vi "Get-selected-motors.vi"(8 "error in (no error)":errorcluster, 11 "Object ref in":T1) -> (0 "error out":errorcluster, 2 "Active?":bool[](array[boolean]), 3 "Object ref out":T1)   [LabVIEW 2013, in "PowderDeposition.lvlib" / "PD-Main.lvclass"]
uses:
  PD-Main.lvclass
  Object-reference.ctl
  PD-Main.lvclass/PD-Main.ctl
  Read Motors-selection.vi
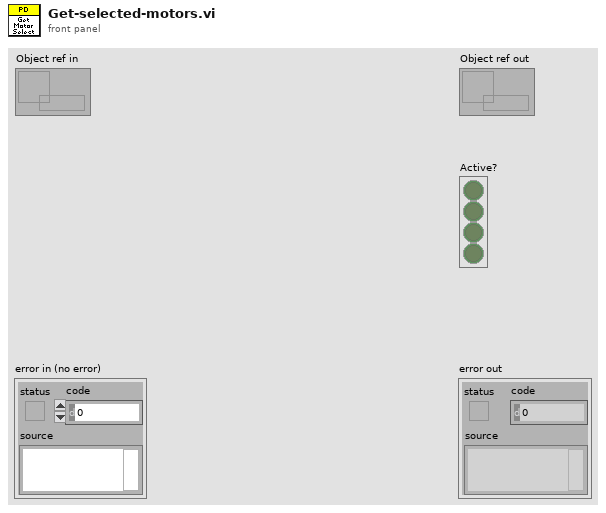
[diagram p1: front panel]
types:
  T1 = typedef "PowderDeposition.lvlib/PD-Main.lvclass/Object-reference.ctl" = refnum<data-value>
  T2 = typedef "PowderDeposition.lvlib/Motor-assembly.lvclass/Motor-selection.ctl" = cluster{"Motor 1":bool, "Motor 2":bool, "Motor 3":bool, "Motor 4":bool}
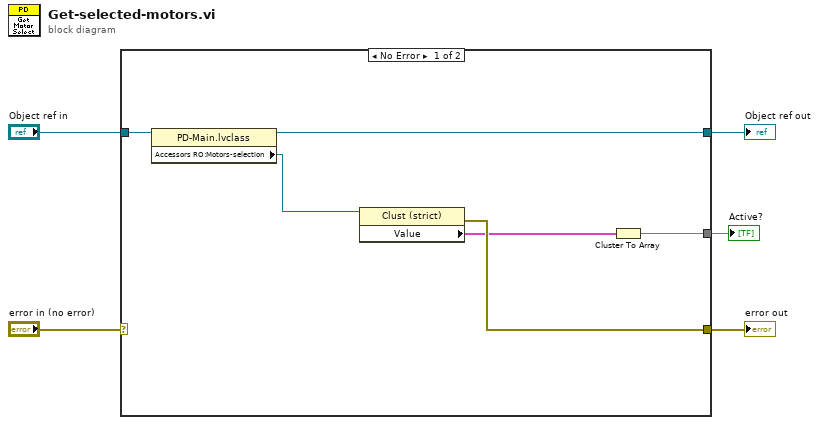
[diagram p0: block diagram]
diagram:
  n1 = case shown="No Error" "error in (no error)" {
    selector: "error in (no error)" -> [_ w13]
    tunnel: [w9 w13] -> w4
    tunnel: [w10 w12] -> w2
    tunnel: "Object ref in" -> [w11 w12]
    tunnel: [w6 _] -> w1
    frame No Error {
      n2 = property class="PD-Main.lvclass"(reference=w11) -> (reference out=w10:T1, "Accessors RO:Motors-selection"=w8:refnum<vi>)  [unwired: 1 in, 1 out]
      n3 = property class="Clust (strict)"(reference=w8) -> (error out=w9:errorcluster, "Value"=w7:T2)  [unwired: 1 in, 1 out]
      n4 = Cluster To Array(cluster=w7) -> (array=w6:bool[])
    }
    frame Error {
    }
  }
  "error out" <- w4
  "Object ref out" <- w2
  "Active?" <- w1
